vi "Ultrasonic new.vi"(6 "Offset X":cluster{"Offset X L":dbl, "Offset X R":dbl}={"Offset X L"=15.0, "Offset X R"=15.0}, 8 "error in (no error)":errorcluster, 11 "Pulse in":T2) -> (0 "error out":errorcluster, 2 "PING":cluster{"PING left":dbl, "PING right":dbl}, 3 "Pulse out":T1)   [LabVIEW 2020]
uses:
  <vilib>/High Genius/HG_WSI_Tookit/Dependencies/Library/Pulse/Pulse.lvclass
  <vilib>/High Genius/HG_WSI_Tookit/Dependencies/Library/ISQ/ISQ.lvclass
  <vilib>/High Genius/HG_WSI_Tookit/Dependencies/Library/VMX Library.lvlib
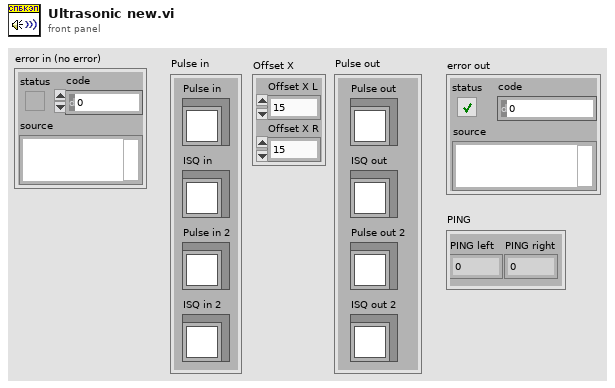
[diagram p1: front panel]
types:
  T1 = cluster{"Pulse out":refnum<class "Pulse.lvclass">, "ISQ out":refnum<class "ISQ.lvclass">, "Pulse out 2":refnum<class "Pulse.lvclass">, "ISQ out 2":refnum<class "ISQ.lvclass">}
  T2 = cluster{"Pulse in":refnum<class "Pulse.lvclass">, "ISQ in":refnum<class "ISQ.lvclass">, "Pulse in 2":refnum<class "Pulse.lvclass">, "ISQ in 2":refnum<class "ISQ.lvclass">}
  T3 = typedef "Semaphore RefNum" = refnum<k1>
  T4 = cluster{"titanenc0":i32, "titanenc1":i32, "titanenc2":i32, "titanenc3":i32, "rpm0":i16, "rpm1":i16, "rpm2":i16, "rpm3":i16, "resetenc0":bool, "resetenc1":bool, "resetenc2":bool, "resetenc3":bool}
  T5 = cluster{"data":cluster{"ai22":sgl, "ai23":sgl, "ai24":sgl, "ai25":sgl, "pulse12":i32, "pulse13":i32, "pwm14":i32, "pwm15":i32, "pwm16":dbl, "do17":bool, "do18":bool, "do19":bool, "do20":bool, "do21":bool, "di11":bool, "di9":bool, "motor0":u8, "motor1":u8, "motor2":u8, "motor3":u8, "dir00":u8, "dir01":u8, "dir02":u8, "dir03":u8, "dir10":u8, "dir11":u8, "dir12":u8, "dir13":u8, "limit0":bool, "limit1":bool, "limit2":bool, "limit3":bool, "limit4":bool, "limit5":bool, "limit6":bool, "limit7":bool, "lsb0H":u8, "lsb1H":u8, "lsb2H":u8, "lsb3H":u8, "lsb0L":u8, "lsb1L":u8, "lsb2L":u8, "lsb3L":u8, "enc0_counters":u32, "enc1_counters":u32, "enc2_counters":u32, "enc3_counters":u32, "counter10":u32, "counter8":u32, "reset_enc0":bool, "reset_enc1":bool, "reset_enc2":bool, "reset_enc3":bool, "pitch":sgl, "roll":sgl, "yaw":sgl, "zero_yaw":bool}}
  T6 = cluster{"data":cluster{"ai22":sgl, "ai23":sgl, "ai24":sgl, "ai25":sgl, "pulse12":i32, "pulse13":i32, "pwm14":i32, "pwm15":i32, "pwm16":i32, "do17":bool, "do18":bool, "do19":bool, "do20":bool, "do21":bool, "di11":bool, "di9":bool, "motor0":u8, "motor1":u8, "motor2":u8, "motor3":u8, "dir00":u8, "dir01":u8, "dir02":u8, "dir03":u8, "dir10":u8, "dir11":u8, "dir12":u8, "dir13":u8, "limit0":bool, "limit1":bool, "limit2":bool, "limit3":bool, "limit4":bool, "limit5":bool, "limit6":bool, "limit7":bool, "lsb0H":u8, "lsb1H":u8, "lsb2H":u8, "lsb3H":u8, "lsb0L":u8, "lsb1L":u8, "lsb2L":u8, "lsb3L":u8, "enc0_counters":u32, "enc1_counters":u32, "enc2_counters":u32, "enc3_counters":u32, "counter10":u32, "counter8":u32, "reset_enc0":bool, "reset_enc1":bool, "reset_enc2":bool, "reset_enc3":bool, "pitch":sgl, "roll":sgl, "yaw":sgl, "zero_yaw":bool}}
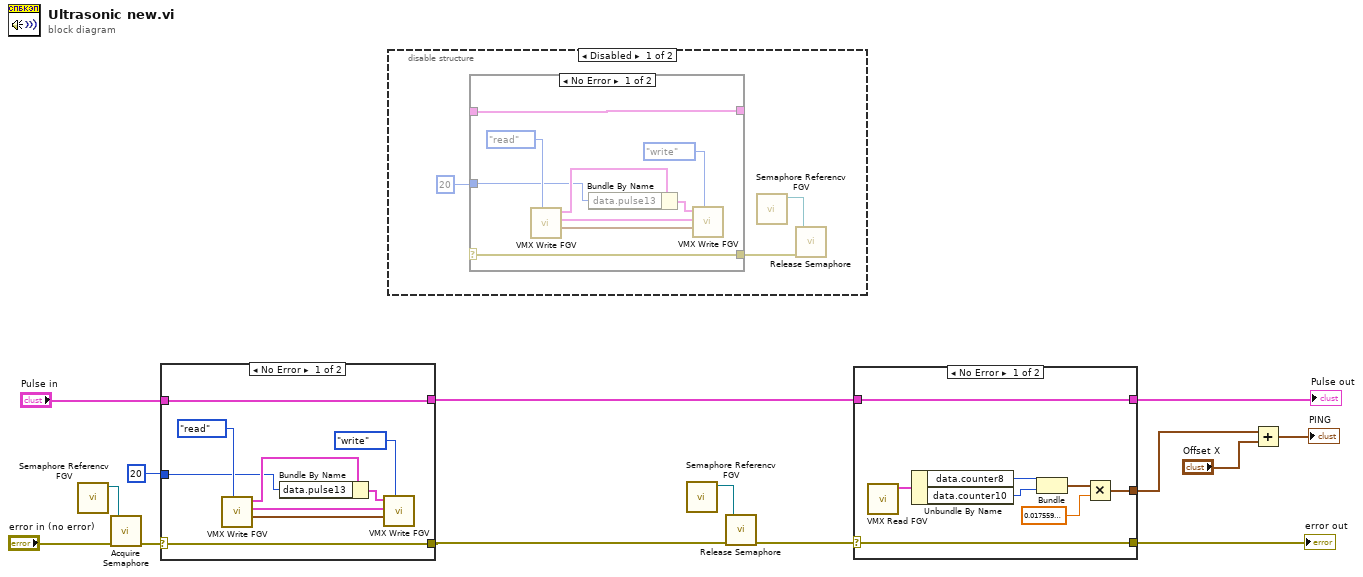
[diagram p0: block diagram]
diagram:
  n1 = call <vilib>:"Semaphore Referencv FGV.vi"() -> ("Semaphore Reference"=w12:T3)  [unwired: 11 in]
  n2 = call <vilib>:"Acquire Semaphore.vi"("error in (no error)"="error in (no error)", "semaphore"=w12) -> ("error out"=w7:errorcluster)  [unwired: 3 in, 2 out]
  n3 = case shown="No Error" w7 {
    selector: w7 -> [w16 w24]
    tunnel: 20 ("Pluse") -> [w15 _]
    tunnel: "Pulse in" -> [w17 w25]
    tunnel: [w17 w25] -> w4
    tunnel: [w16 w24] -> w2
    frame No Error {
      n4 = call <vilib>:"VMX Write FGV.vi"("Enum"=enum16{"read", "write"}."read") -> ("Read Data3"=w21:cluster{"pwm17":i32, "pwm18":i32}, "Read Data2"=w20:T4, "Read Data"=w19:T5)  [unwired: 8 in]
      n5 = Bundle By Name(cluster=w19, "data.pulse13"=w15) -> (w18:T5)
      n6 = call <vilib>:"VMX Write FGV.vi"("Enum"=enum16{"read", "write"}."write", "Write Data3"=w21, "Write Data2"=w20, "Write Data"=w18) -> ()  [unwired: 5 in, 3 out]
    }
    frame Error {
    }
  }
  n7 = disable-structure shown="Disabled" {
    frame Disabled {
      n8 = case shown="No Error" {
        selector: _ -> [w30 w38]
        tunnel: 20 ("Pluse") -> [w29 _]
        tunnel: _ -> [w31 w39]
        tunnel: [w31 w39] -> _
        tunnel: [w30 w38] -> w26
        frame No Error {
          n9 = call <vilib>:"VMX Write FGV.vi"("Enum"=enum16{"read", "write"}."read") -> ("Read Data3"=w35:cluster{"pwm17":i32, "pwm18":i32}, "Read Data2"=w34:T4, "Read Data"=w33:T5)  [unwired: 8 in]
          n10 = Bundle By Name(cluster=w33, "data.pulse13"=w29) -> (w32:T5)
          n11 = call <vilib>:"VMX Write FGV.vi"("Enum"=enum16{"read", "write"}."write", "Write Data3"=w35, "Write Data2"=w34, "Write Data"=w32) -> ()  [unwired: 5 in, 3 out]
        }
        frame Error {
        }
      }
      n12 = call <vilib>:"Semaphore Referencv FGV.vi"() -> ("Semaphore Reference"=w27:T3)  [unwired: 11 in]
      n13 = call <vilib>:"Release Semaphore.vi"("error in (no error)"=w26, "semaphore"=w27) -> ()  [unwired: 4 in, 2 out]
    }
    frame Enabled {
    }
  }
  n14 = call <vilib>:"Semaphore Referencv FGV.vi"() -> ("Semaphore Reference"=w3:T3)  [unwired: 11 in]
  n15 = call <vilib>:"Release Semaphore.vi"("error in (no error)"=w2, "semaphore"=w3) -> ("error out"=w1:errorcluster)  [unwired: 4 in, 1 out]
  n16 = case shown="No Error" w1 {
    selector: w1 -> [w46 w48]
    tunnel: w4 -> [w47 w49]
    tunnel: [w47 w49] -> w10
    tunnel: [w46 w48] -> w9
    tunnel: [w40 _] -> w8
    frame No Error {
      n17 = call <vilib>:"VMX Read FGV.vi"() -> ("Read Data"=w45:T6)  [unwired: 10 in, 1 out]
      n18 = Unbundle By Name(w45) -> ("data.counter8"=w44:u32, "data.counter10"=w43:u32)
      n19 = Bundle("counter8"=w44, "counter10"=w43) -> (w42:cluster{"counter8":u32, "counter10":u32})  [unwired: 1 in]
      n20 = Multiply(x=w42, y=sgl 0.01756) -> (x*y=w40:cluster{"counter8":sgl, "counter10":sgl})
    }
    frame Error {
    }
  }
  "error out" <- w9
  "Pulse out" <- w10
  n21 = Add(x=w8, y="Offset X") -> (x+y=→"PING":cluster{dbl, dbl})
